vi "ActionVIOnCompile.vi"(8 "error in (no error)":errorcluster, 11 "Device Item Ref in":T1 format="%.0x") -> (0 "error out":errorcluster)   [LabVIEW 2018, in "CAN Gateway System Explorer.lvlib"]
uses:
  CAN Gateway System Explorer.lvlib
  <vilib>/NI Veristand/Custom Device API/Custom Device Item Ref.ctl
  Shared/CTLs/Compiled Data.ctl
  Shared/CTLs/Corruption Info.ctl
  Shared/CTLs/Frame.ctl
  Shared/CTLs/Signal_Data_Trigger.ctl
  Types/FrameDirection.ctl
  Shared/Constants.vi
  <vilib>/NI Veristand/Custom Device API/Set Item Property (Variant).vi
  <vilib>/NI Veristand/Custom Device API/Custom Device API.lvlib
  Shared/CAN Gateway Shared.lvlib
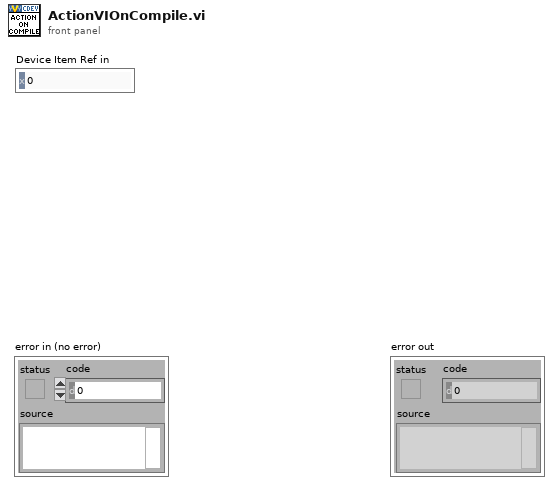
[diagram p1: front panel]
types:
  T1 = typedef "Custom Device API.lvlib/Custom Device Item Ref.ctl" = u64
  T2 = typedef "CAN Gateway System Explorer.lvlib/FrameDirection.ctl" = enum16{"NET_TO_DUT", "DUT_TO_NET"}
  T3 = typedef "CAN Gateway Shared.lvlib/Compiled Data.ctl" = cluster{"HW Info Network Port":cluster{"CAN Port":string, "Baudrate":u64}, "HW Info DUT Port":cluster{"CAN Port":string, "Baudrate":u64}, "Corruption Info Network_DUT":T4, "Corruption Info DUT_Network":T4}
  T4 = typedef "CAN Gateway Shared.lvlib/Corruption Info.ctl" = cluster{"Corrupt IDs Array":u32[], "Frame Infos Array":T5[]}
  T5 = typedef "CAN Gateway Shared.lvlib/Frame.ctl" = cluster{"Disable Frame Channel Index":i32, "Has  CRC?":bool, "CRC start Bit":u32, "DLC corruption Channel Index":i32, "DLC Length  Corruption Index":i32, "CRC Index":i32, "Conversion Session":refnum<k21>, "CRC Signal":refnum<k21>, "Data Signal Array":T6[]}
  T6 = typedef "CAN Gateway Shared.lvlib/Signal_Data_Trigger.ctl" = cluster{"XNET Signal":refnum<k21>, "Data Idx":u32, "Trigger Idx":u32}
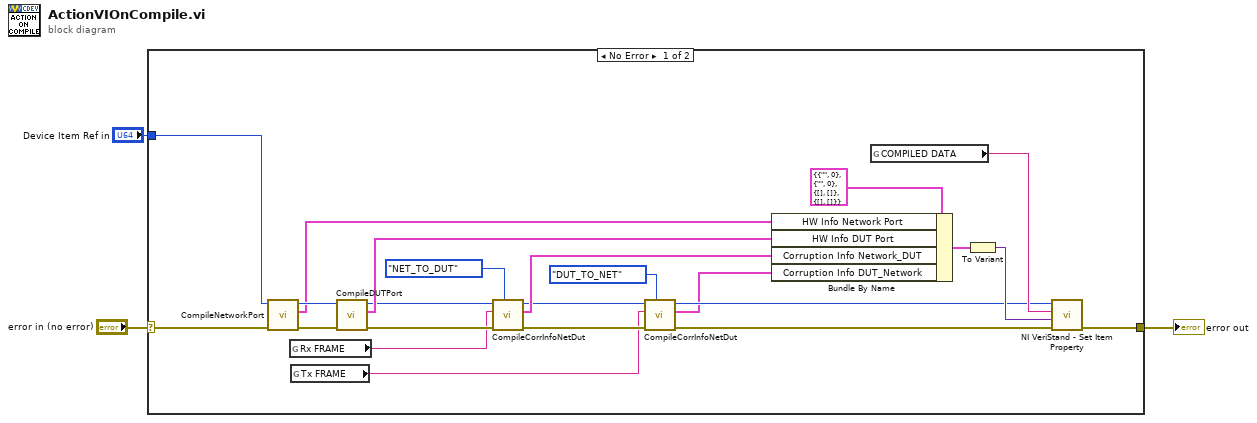
[diagram p0: block diagram]
diagram:
  n1 = case shown="No Error" "error in (no error)" {
    selector: "error in (no error)" -> [w5 w27]
    tunnel: [w26 w27] -> w2
    tunnel: "Device Item Ref in" -> [w4 _]
    frame No Error {
      n2 = call "CompileNetworkPort.vi"("error in (no error)"=w5, "Device Item Ref in"=w4) -> ("error out"=w21:errorcluster, "HW Info DUT Port"=w19:cluster{"CAN Port":string, "Baudrate":u64}, "Device Item Ref out"=w20:T1)  [unwired: 7 in]
      n3 = global read "Constants.vi" "Rx FRAME"() -> (w9:string)
      n4 = global read "Constants.vi" "Tx FRAME"() -> (w8:string)
      n5 = call "CompileDUTPort.vi"("error in (no error)"=w21, "Device Item Ref in"=w20) -> ("error out"=w17:errorcluster, "HW Info DUT Port"=w18:cluster{"CAN Port":string, "Baudrate":u64}, "Device Item Ref out"=w16:T1)  [unwired: 7 in]
      n6 = call "CompileCorrInfoNetDut.vi"("Frame Direction"=FrameDirection."NET_TO_DUT", "error in (no error)"=w17, "Frame Direction Prop"=w9, "Device Item Ref in"=w16) -> ("error out"=w10:errorcluster, "Corruption Info Network_DUT"=w15:T4, "Device Item Ref out"=w14:T1)  [unwired: 5 in]
      n7 = call "CompileCorrInfoNetDut.vi"("Frame Direction"=FrameDirection."DUT_TO_NET", "error in (no error)"=w10, "Frame Direction Prop"=w8, "Device Item Ref in"=w14) -> ("error out"=w13:errorcluster, "Corruption Info Network_DUT"=w11:T4, "Device Item Ref out"=w12:T1)  [unwired: 5 in]
      n8 = Bundle By Name(cluster=T3 {"HW Info Network Port"={"CAN Port"="", "Baudrate"=0}, "HW Info DUT Port"={"CAN Port"="", "Baudrate"=0}, "Corruption Info Network_DUT"={"Corrupt IDs Array"=[], "Frame Infos Array"=[]}, "Corruption Info DUT_Network"={"Corrupt IDs Array"=[], "Frame Infos Array"=[]}} ("Compiled Data"), "HW Info Network Port"=w19, "HW Info DUT Port"=w18, "Corruption Info Network_DUT"=w15, "Corruption Info DUT_Network"=w11) -> (w22:T3)
      n9 = global read "Constants.vi" "COMPILED DATA"() -> (w25:string)
      n10 = To Variant(anything=w22) -> (Variant=w24:variant)
      n11 = call-poly <vilib>:"NI VeriStand - Set Item Property.vi"("error in (no error)"=w13, "Value"=w24, "Property Name"=w25, "Item Ref in"=w12) -> ("error out"=w26:errorcluster)  [unwired: 5 in, 2 out]
    }
    frame Error {
    }
  }
  "error out" <- w2
